vi "pie sbv.vi"(8 "s":bool, 9 "rect 2":T1, 10 "Next 1?":bool, 11 "Height":u32) -> (2 "rect":T1)   [LabVIEW 2019, in "Zen Analytics.lvlib" / "Zen Analytics.lvclass"]
uses:
  Zen Analytics.lvclass
types:
  T1 = cluster{"left":i16, "top":i16, "right":i16, "bottom":i16}
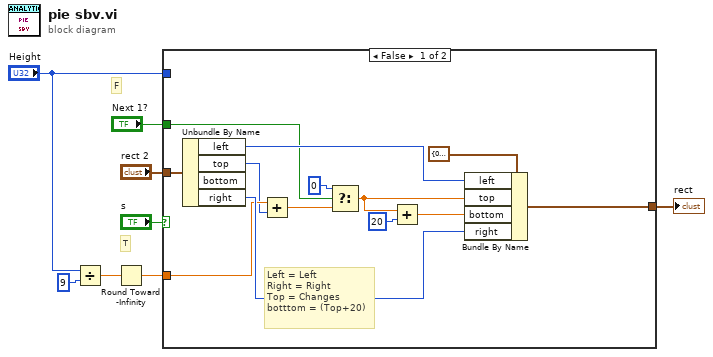
[diagram p0: block diagram]
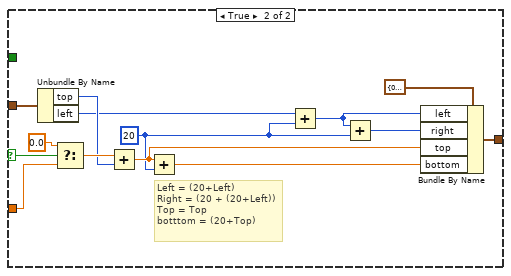
[diagram p2: hidden frame]
diagram:
  # "F"
  # "T"
  n1 = Divide(x="Height", y=9 ("Array Size")) -> (x/y=w7:dbl)
  n2 = Round Toward -Infinity(1:w7) -> (0:w5:dbl)
  n3 = case shown="False" "s" {
    selector: "s" -> [_ w35]
    tunnel: w5 -> [w14 w33]
    tunnel: "Height" -> [_ _]
    tunnel: "rect 2" -> [w21 w30]
    tunnel: [w15 w27] -> w3
    tunnel: "Next 1?" -> [w12 _]
    frame False {
      # "Left = Left\nRight = Right\nTop = Changes\nbotttom = (Top+20)"
      n4 = Unbundle By Name(w21) -> ("left"=w20:i16, "top"=w13:i16, "right"=w18:i16)  [unwired: 1 out]
      n5 = Add(x=w14, y=w13) -> (x+y=w10:dbl)
      n6 = Select(t=i16 0 ("y"), s=w12, f=w10) -> (s? t:f=w9:dbl)
      n7 = Add(x=w9, y=i16 20) -> (x+y=w17:dbl)
      n8 = Bundle By Name(cluster=T1 {"left"=0, "top"=0, "right"=0, "bottom"=0} ("rect 2"), "left"=w20, "top"=w9, "bottom"=w17, "right"=w18) -> (w15:T1)
    }
    frame True {
      w23 = 20
      # "Left = (20+Left)\nRight = (20 + (20+Left))\nTop = Top\nbotttom = (20+Top)"
      n9 = Unbundle By Name(w30) -> ("top"=w28:i16, "left"=w22:i16)
      n10 = Select(t=0.0, s=w35, f=w33) -> (s? t:f=w29:dbl)
      n11 = Add(x=w29, y=w28) -> (x+y=w25:dbl)
      n12 = Add(x=w25, y=w23) -> (x+y=w24:dbl)
      n13 = Add(x=w22, y=w23) -> (x+y=w32:i32)
      n14 = Add(x=w32, y=w23) -> (x+y=w31:i32)
      n15 = Bundle By Name(cluster=T1 {"left"=0, "top"=0, "right"=0, "bottom"=0} ("rect 2"), "left"=w32, "right"=w31, "top"=w25, "bottom"=w24) -> (w27:T1)
    }
  }
  "rect" <- w3
